vi "SAOMM-XMLNodeParser.vi"(5 "NodeName":string[](array[string]), 9 "Node Text":string[](array[string])) -> (8 "PointData":dbl[](array[numeric]) format="%.6f")   [LabVIEW 2019]
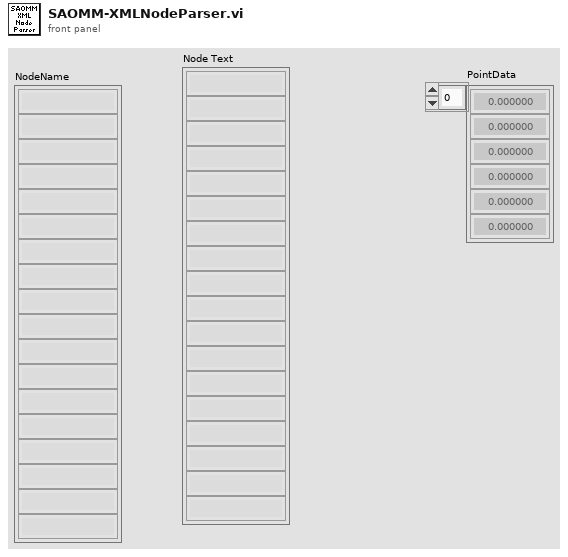
[diagram p1: front panel]
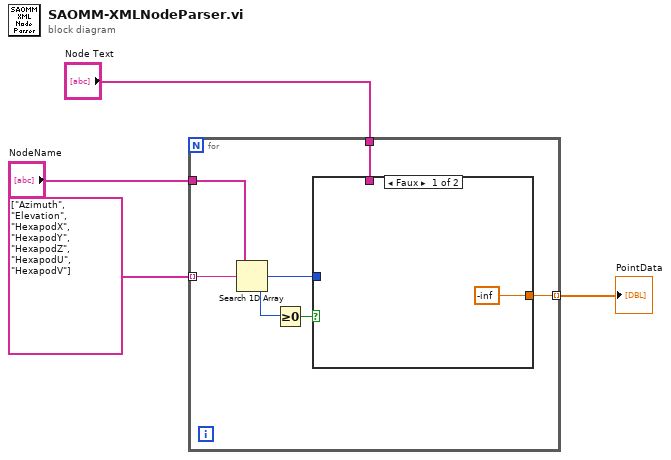
[diagram p0: block diagram]
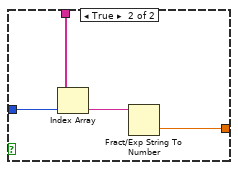
[diagram p2: hidden frame]
diagram:
  n1 = for {
    tunnel: "NodeName" -> [w9]
    tunnel: string[] ["Azimuth", "Elevation", "HexapodX", "HexapodY", "HexapodZ", "HexapodU", "HexapodV"] -> [w10] mode=indexing
    tunnel: "Node Text" -> [w8]
    tunnel: [w5] -> w1 mode=indexing
    n2 = Search 1D Array(1D array=w9, element=w10) -> (index of element=w6:i32)  [unwired: 1 in]
    n3 = Greater Or Equal To 0?(x=w6) -> (x >= 0?=w7:bool)
    n4 = case shown="Faux" w7 {
      tunnel: w6 -> [_ w15]
      tunnel: w8 -> [_ w14]
      tunnel: [-inf w12] -> w5
      frame False {
      }
      frame True {
        n5 = Index Array(array=w14, index=w15) -> (element=w13:string)
        n6 = Fract/Exp String To Number(string=w13) -> (number=w12:dbl)  [unwired: 3 in, 1 out]
      }
    }
  }
  "PointData" <- w1
